vi "Navigation_Main_derping_stuff_up april 14_2.vi"() -> ()   [LabVIEW 2015]
uses:
  <vilib>/myRIO/Instrument Drivers/Onboard IO/PWM/typedefs/PWM Reference.ctl
  <vilib>/myRIO/Common/Instrument Driver Framework/Utilities/typedefs/myRIO Generic Hardware Reference.ctl
  <vilib>/myRIO/Common/Instrument Driver Framework/Utilities/typedefs/Hardware Version Enum.ctl
  <vilib>/myRIO/Common/Instrument Driver Framework/Utilities/typedefs/myRIO v1.0 Reference.ctl
  <vilib>/myRIO/Common/Instrument Driver Framework/Utilities/typedefs/Generic FPGA Reference.ctl
  <vilib>/myRIO/Common/Instrument Driver Framework/myRIO v1.0/PWM/typedefs/PWM Channels Enum.ctl
  <vilib>/myRIO/Instrument Drivers/Onboard IO/PWM/typedefs/PWM Configuration.ctl
  <vilib>/userdefined/High Color/nirio_resource_hc.ctl
  <vilib>/myRIO/Common/Instrument Driver Framework/myRIO v1.0/PWM/vis/myRIO v1.1 Open PWM.vi
  <vilib>/myRIO/Common/Instrument Driver Framework/Utilities/vis/Validate Channels.vi
  <vilib>/myRIO/Common/Instrument Driver Framework/myRIO v1.0/PWM/vis/myRIO v1.0 Reserve PWM.vi
  <vilib>/myRIO/Common/Instrument Driver Framework/myRIO v1.0/PWM/vis/myRIO v1.0 Build MUX Configuration PWM.vi
  <vilib>/myRIO/Common/Instrument Driver Framework/myRIO v1.0/Resource Manager/vis/myRIO v1.0 Reserve Channel List.vi
  <vilib>/myRIO/Common/Instrument Driver Framework/myRIO v1.0/Resource Manager/vis/myRIO v1.0 Create Configuration List.vi
  <vilib>/myRIO/Common/Instrument Driver Framework/myRIO v1.0/Resource Manager/vis/myRIO v1.0 Reserve Channel.vi
  <vilib>/myRIO/Common/Instrument Driver Framework/myRIO v1.0/Resource Manager/vis/myRIO v1.0 Unreserve Channel.vi
  <vilib>/myRIO/Common/Instrument Driver Framework/myRIO v1.0/Resource Manager/vis/myRIO v1.0 Build Mutex Name.vi
  <vilib>/FPGAPlugInAG/myRIO-1900/niLvFpga_Open_myRIO-1900.vi
  <vilib>/rvi/interface/common/dynamic/niFpgaDynamicAddResources.vi
  <vilib>/myRIO/Common/Instrument Driver Framework/Utilities/vis/FPGA Ref Manager.vi
  <vilib>/Utility/error.llb/Error Cluster From Error Code.vi
  <vilib>/myRIO/Common/Instrument Driver Framework/Utilities/vis/Ref Counter.vi
  <vilib>/rvi/errors/niLvFpgaAdjustHostInterfaceError.vi
  <vilib>/Utility/VariantDataType/GetNumericInfo.vi
  <vilib>/myRIO/Common/Instrument Driver Framework/myRIO v1.0/myRIO v1.1 Open.vi
  <vilib>/myRIO/Common/Instrument Driver Framework/Utilities/vis/IO Manager.vi
  <vilib>/myRIO/Common/Instrument Driver Framework/Utilities/vis/Configuration Manager.vi
  <vilib>/myRIO/Common/Instrument Driver Framework/myRIO v1.0/Resource Manager/vis/myRIO v1.0 Configure IO.vi
  <vilib>/myRIO/Common/Instrument Driver Framework/myRIO v1.0/myRIO v1.0 Close.vi
  <vilib>/myRIO/Common/Instrument Driver Framework/myRIO v1.0/PWM/vis/myRIO v1.0 Write PWM.vi
  <vilib>/addons/control/pid/pid.llb/PID (DBL).vi
  <vilib>/rvi/interface/nirviOpenFPGA/nirviOpenFPGA.xnode
  Navi/E/FPGA Bitfiles/NavigationProjec_FPGATarget2_FPGAMainNavigati_PWPHW8gwDxI.lvbitx
  <vilib>/rvi/interface/nirviReadWriteControl/nirviReadWriteControl.xnode
  <vilib>/myRIO/Instrument Drivers/Onboard IO/PWM/vis/myRIO PWM Open.xnode
  <vilib>/myRIO/Instrument Drivers/Onboard IO/PWM/PWM.lvlib
  <vilib>/myRIO/Instrument Drivers/Utilities/Utilities.lvlib
  NiFpgaLv.dll
  <vilib>/rvi/interface/Simulation/niFpgaSimulationCallBeginRW.vi
  <vilib>/addons/control/pid/NI_PID_pid.lvlib
panel:
  out "stop switch":dbl=1.0
  out "distance to goal":dbl
  out "loc_y":dbl
  out "loc_x":dbl
  out "loc_theta":dbl
  out "start y":dbl
  out "start angle":dbl=1.0
  out "start x":dbl=1.0
  in  "set start position":bool=TRUE
  out "goal reached":bool=TRUE
  out "x/y":dbl
  out "scale":dbl=1.0
  in  "x goal":dbl=10.0
  in  "L Desired Input Velocity (ft/s) 4":dbl(knob) scale=-4.0..4.0
  in  "R Min Linear Velocity (ft/s)  2":dbl=-2.0 format="%#_13g"
  in  "L Min Linear Velocity (ft/s) 9":dbl=-2.0 format="%#_13g"
  in  "R Max Linear Velocity (ft/s) 5":dbl=2.0 format="%#_13g"
  in  "L Max Linear Velocity (ft/s) 5":dbl=2.0 format="%#_13g"
  in  "R Desired Input Velocity (ft/s) 5":dbl(knob) scale=-4.0..4.0
  out "left":dbl
  out "right":dbl
  out "left wheels actual pwm":dbl
  in  "stop 3":bool
  out "left pwm":dbl(graph)
  out "dt out (s) 3":dbl format="%.3f"
  in  "output range 3":cluster{"output high":dbl, "output low":dbl}={"output high"=0.13333, "output low"=-0.13333} {"output low" format="%.6f"; "output high" format="%.5f"}
  in  "PID gains 3":T1={"proportional gain (Kc)"=0.002, "integral time (Ti, min)"=7e-07, "derivative time (Td, min)"=0.0} {"derivative time (Td, min)" format="%.8f"; "integral time (Ti, min)" format="%.8f"; "proportional gain (Kc)" format="%.8f"}
  out "desired pwm 2":dbl
  out "feedback 2":dbl
  out ".not. x? 3":bool
  out "Elapsed Time (s) 2":dbl caption="Elapsed Time (s)"
  out "x traveled 2":dbl
  out "y traveled 2":dbl
  out "avg 124":dbl
  out "avg 457":dbl
  out "psi dot 2":dbl
  out "distance traveled 2":dbl
  out "y dot 2":dbl
  out "x dot 2":dbl
  out "x position 2":dbl
  out "y position 2":dbl
  out "reset x y 2":dbl
  out "Tick Count(mSec) 2":u32 caption="Tick Count(mSec)"
  in  "start y 2":dbl=3.0
  in  "start x 2":dbl=1.0
  out "right wheels actual pwm":dbl
  in  "stop 2":bool
  out "right pwm":dbl(graph)
  out "dt out (s) 2":dbl format="%.3f"
  in  "output range 2":cluster{"output high":dbl, "output low":dbl}={"output high"=0.13333, "output low"=-0.13333} {"output low" format="%.6f"; "output high" format="%.5f"}
  in  "PID gains 2":T1={"proportional gain (Kc)"=0.002, "integral time (Ti, min)"=7e-07, "derivative time (Td, min)"=0.0} {"derivative time (Td, min)" format="%.8f"; "integral time (Ti, min)" format="%.8f"; "proportional gain (Kc)" format="%.8f"}
  out "desired pwm":dbl
  out "feedback":dbl
  out ".not. x? 2":bool
  out "Elapsed Time (s)":dbl
  out "LF Rot Velocity (rot/s)":dbl
  out "LM Rot Velocity (rot/s)":dbl
  out "LR Rot Velocity (rot/s)":dbl
  out "RR Rot Velocity (rot/s)":dbl
  out "RM Linear Velocity (rot/s)":dbl
  out "RF Linear Velocity (rot/s)":dbl
  in  "Encoder Reset":bool
  out "SYS.SELECTA":u8 format="%08b"
  out "ENC.B_c.CNTR":i32
  out "ENC.B_b.CNTR":i32
  out "ENC.B_a.CNTR":i32
  out "ENC.A_c.CNTR":i32
  out "ENC.A_b.CNTR":i32
  out "ENC.A_a.CNTR":i32
  in  "R Min Linear Velocity (ft/s)":dbl=-2.0 format="%#_13g"
  in  "R Max Linear Velocity (ft/s)":dbl=2.0 format="%#_13g"
  in  "L Min Linear Velocity (ft/s)":dbl=-2.0 format="%#_13g"
  in  "L Max Linear Velocity (ft/s)":dbl=2.0 format="%#_13g"
  out "Current Rot Velocity (rot/s)":T2(graph)
  # "Motor Control Parameters"
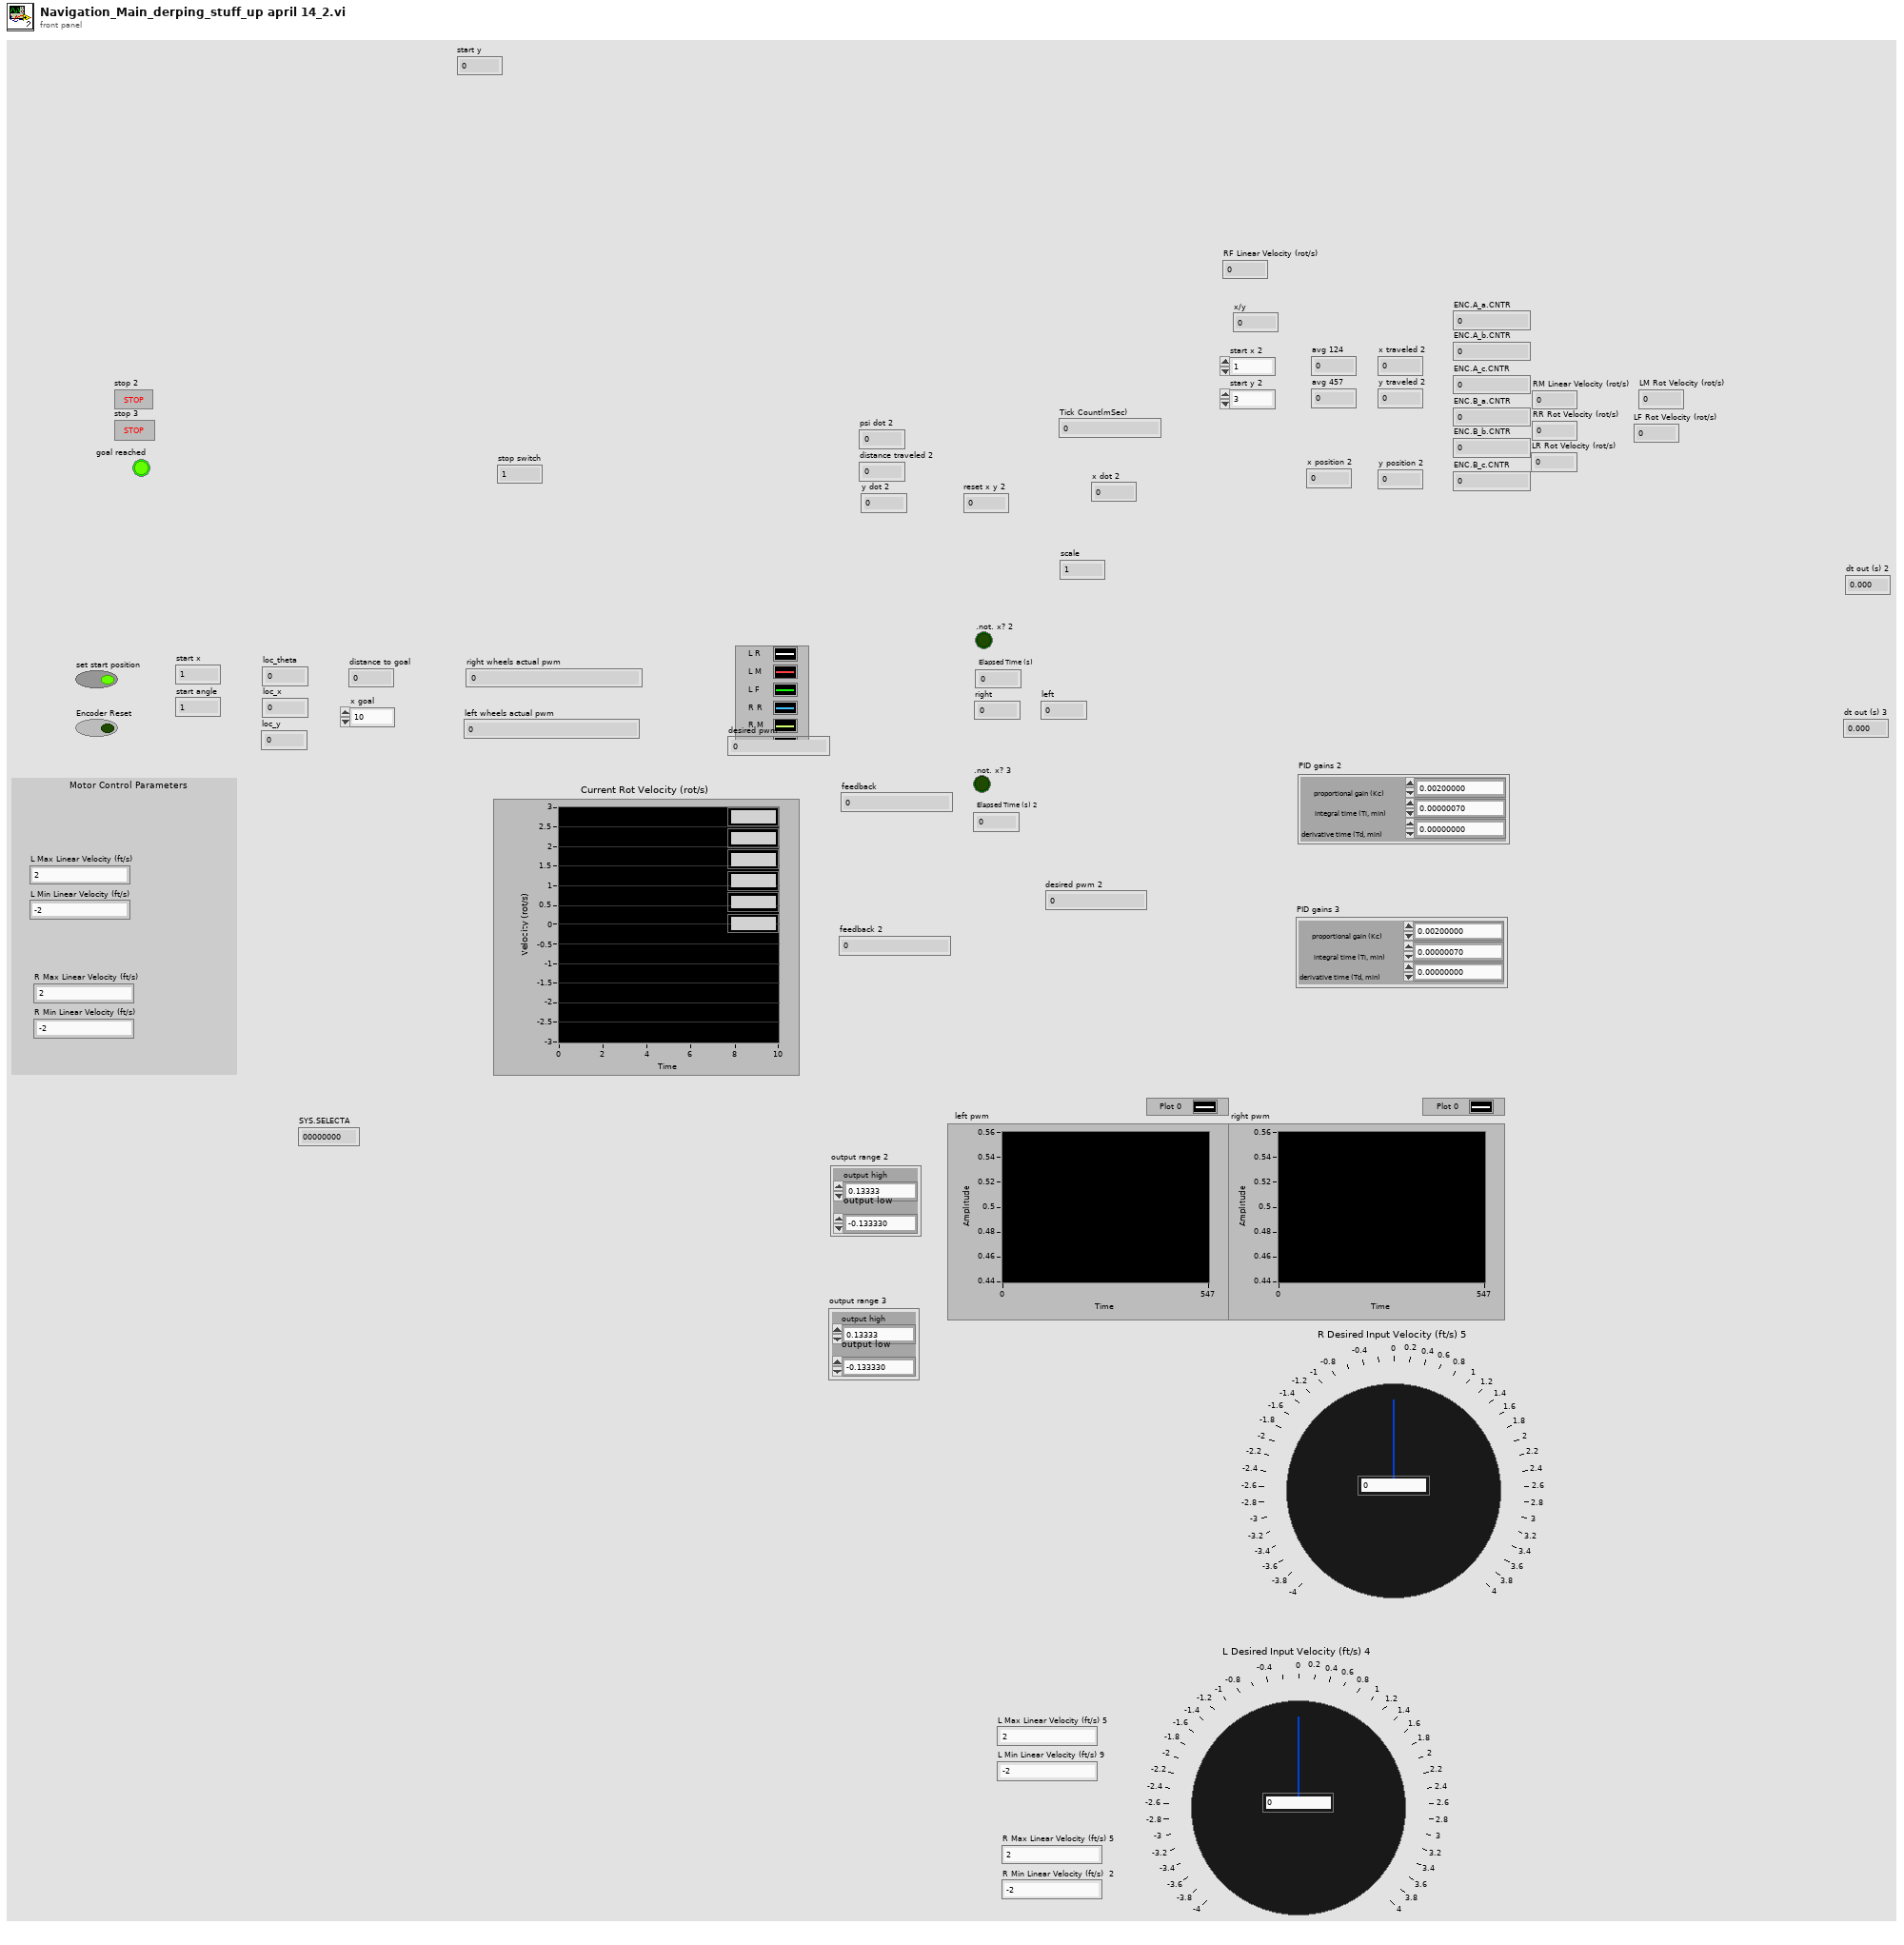
[diagram p1: front panel]
types:
  T1 = cluster{"proportional gain (Kc)":dbl, "integral time (Ti, min)":dbl, "derivative time (Td, min)":dbl}
  T2 = cluster{"Rotational Velocity (RPS)":dbl, "Rotational Velocity (RPS)":dbl, "Rotational Velocity (RPS)":dbl, "Rotational Velocity (RPS)":dbl, "Rotational Velocity (RPS)":dbl, "Rotational Velocity (RPS)":dbl}
  T3 = typedef "nirio_resource_hc.ctl" = tag
  T4 = typedef "Hardware Version Enum.ctl" = enum16{"Unknown", "myRIO-1900", "myRIO-1950", "roboRIO"}
  T5 = typedef "PWM.lvlib/PWM Reference.ctl" = cluster{"myRIO Reference":T6, "PWM Channels Enum":T9, "PWM Configuration":T10}
  T6 = typedef "myRIO Generic Hardware Reference.ctl" = cluster{"myRIO Model":T4, "myRIO Hardware Reference":T7}
  T7 = typedef "myRIO v1.0 Reference.ctl" = cluster{"Generic FPGA Reference":T8, "Allow multiple opens":bool}
  T8 = typedef "Generic FPGA Reference.ctl" = refnum<k20>
  T9 = typedef "PWM Channels Enum.ctl" = enum16{"Not Connected", "C/PWM0", "C/PWM1", "A/PWM0", "A/PWM1", "A/PWM2", "B/PWM0", "B/PWM1", "B/PWM2", "PWM/PWM0", "PWM/PWM1", "PWM/PWM2", "PWM/PWM3", "PWM/PWM4", "PWM/PWM5", "PWM/PWM6", "PWM/PWM7", "PWM/PWM8", "PWM/PWM9"}
  T10 = typedef "PWM.lvlib/PWM Configuration.ctl" = cluster{"Frequency":dbl, "Duty Cycle":dbl}
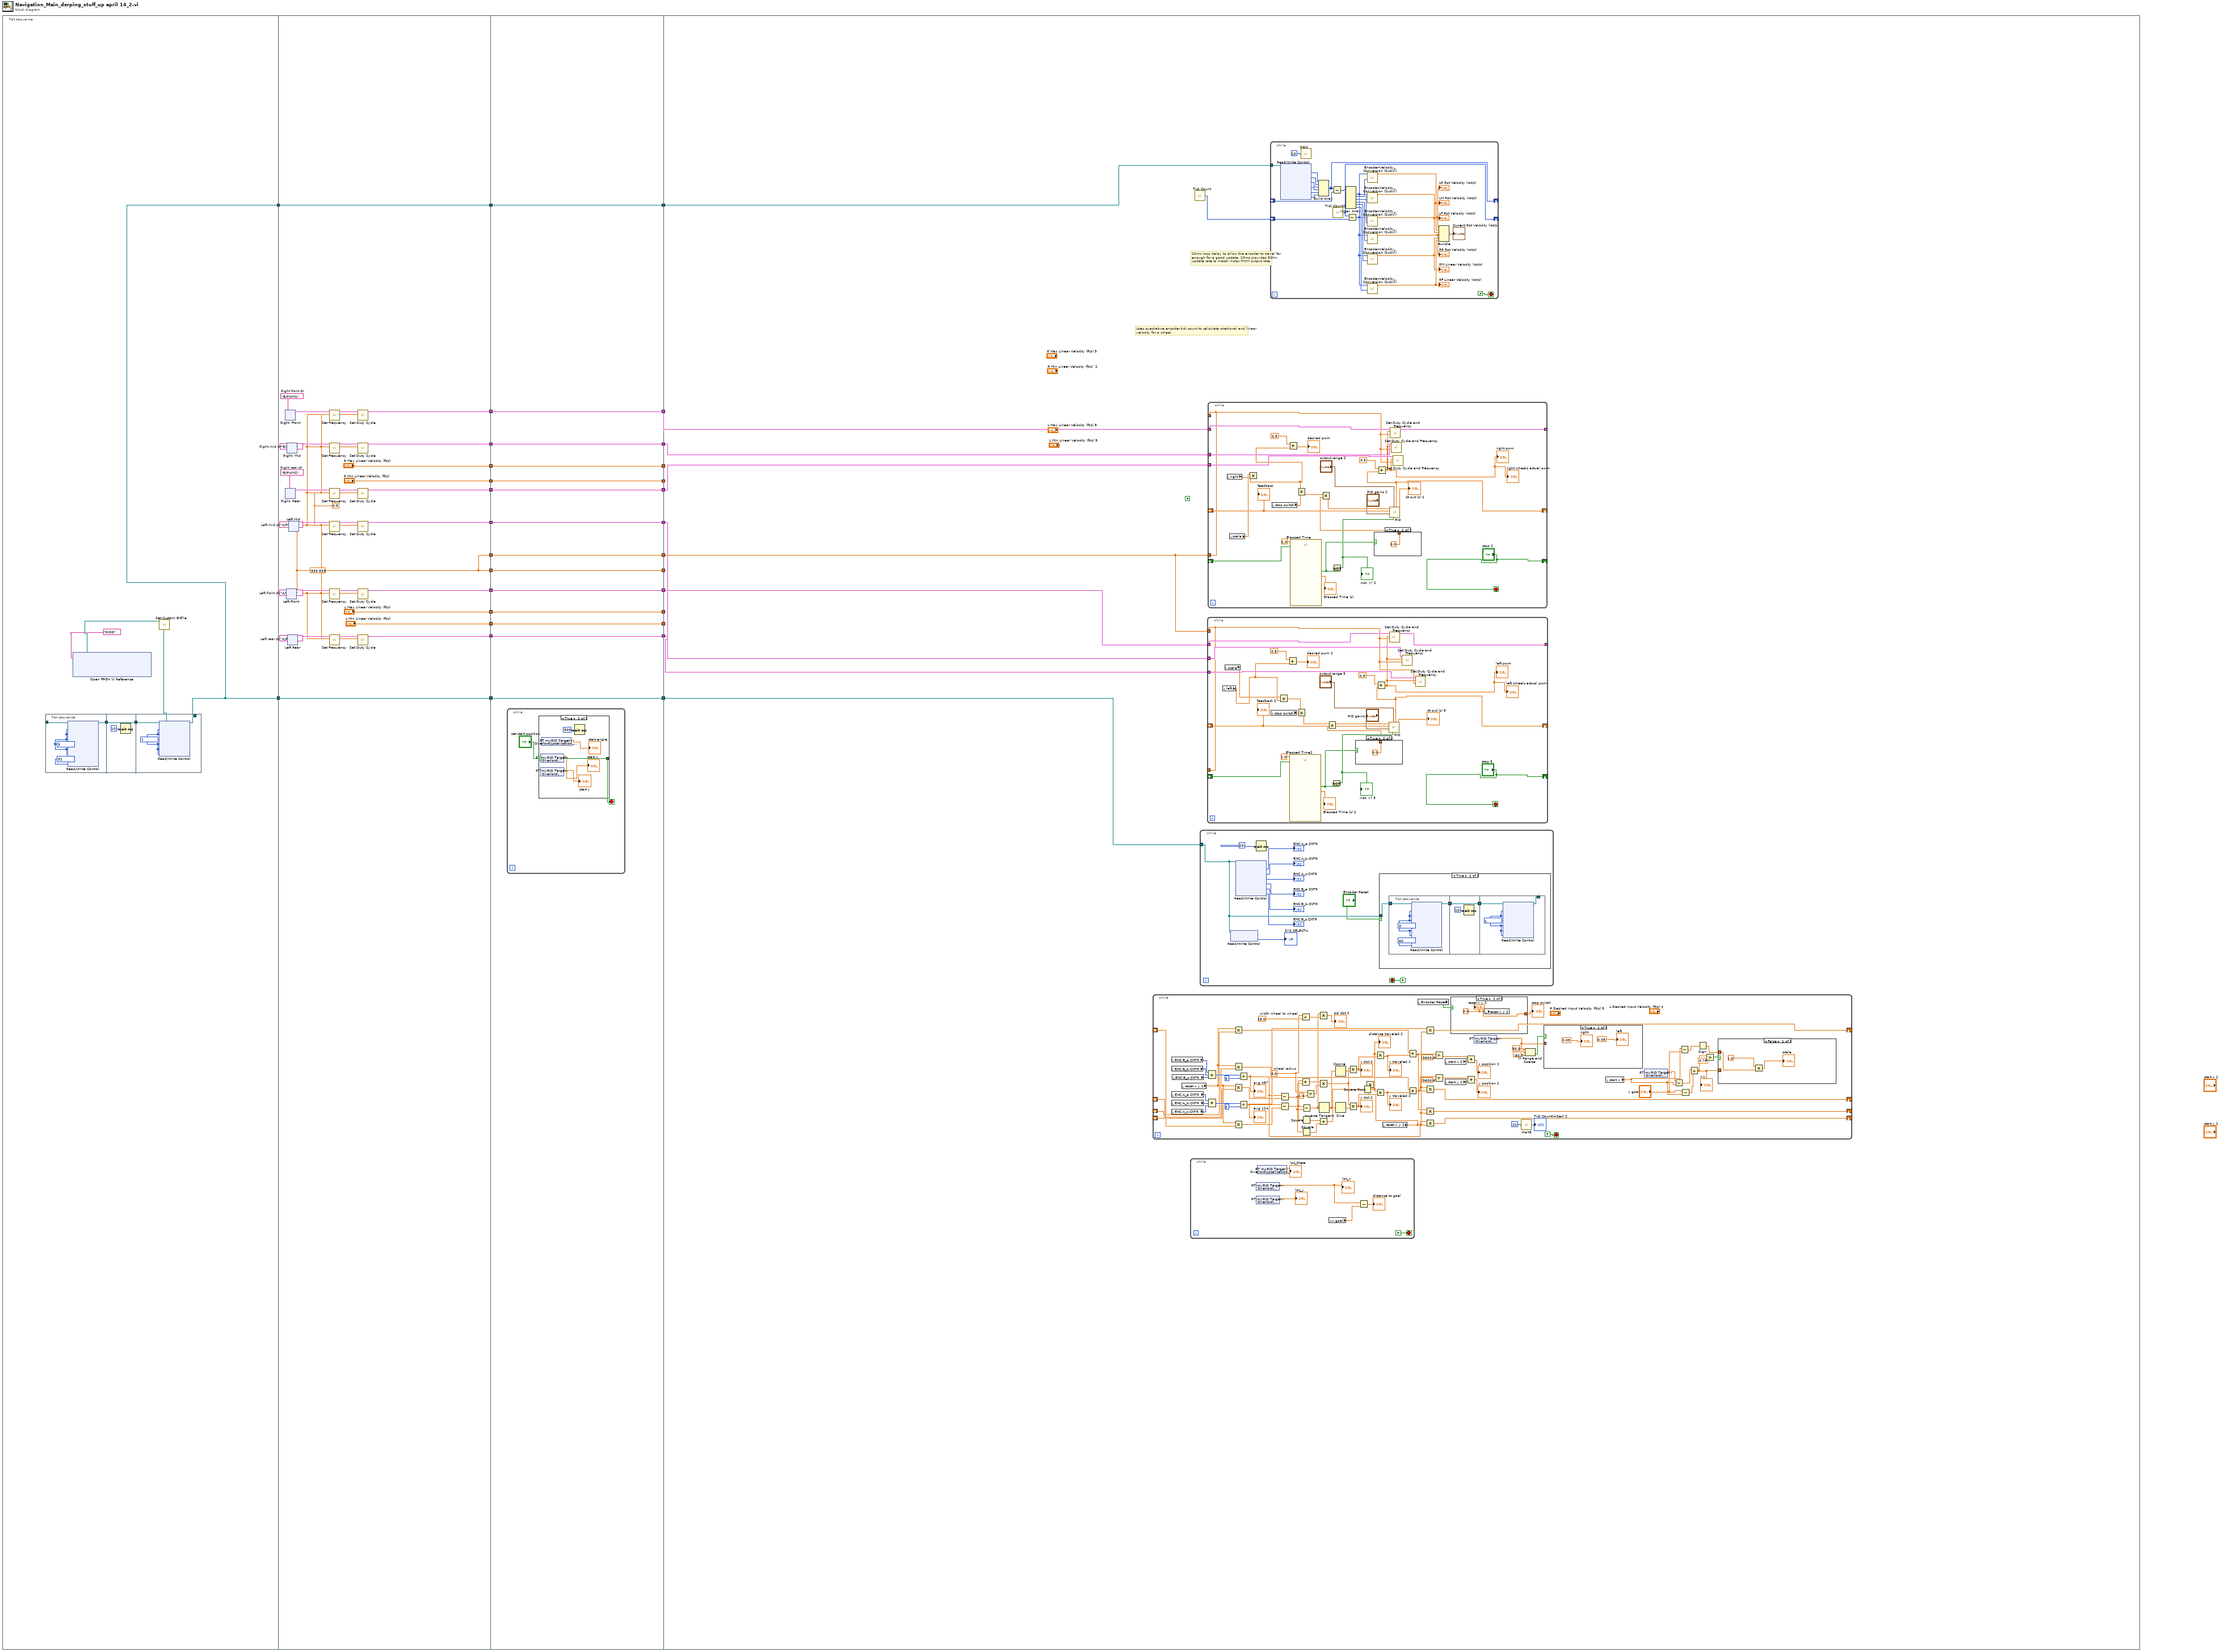
[diagram p0: block diagram]
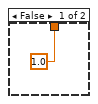
[diagram p3: hidden frame]
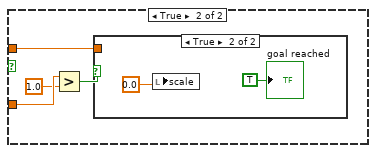
[diagram p4: hidden frame]
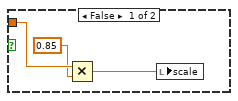
[diagram p5: hidden frame]
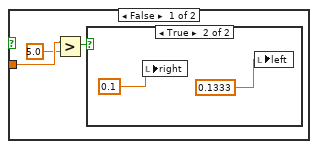
[diagram p6: hidden frame]
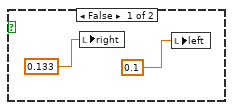
[diagram p7: hidden frame]
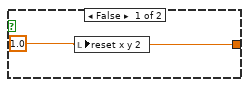
[diagram p8: hidden frame]
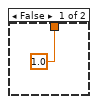
[diagram p9: hidden frame]
diagram:
  n1 = flat-sequence {
    tunnel: [w33] -> w30
    tunnel: [w33] -> w29
    tunnel: [w46] -> w28
    tunnel: [w61] -> w26
    tunnel: [w57] -> w24
    tunnel: [w56] -> w22
    tunnel: [w55] -> w20
    tunnel: [w54] -> w18
    tunnel: [w53] -> w16
    tunnel: ["L Max Linear Velocity (ft/s)"] -> w14
    tunnel: ["L Min Linear Velocity (ft/s)"] -> w12
    tunnel: ["R Max Linear Velocity (ft/s)"] -> w10
    tunnel: ["R Min Linear Velocity (ft/s)"] -> w8
    tunnel: [w48] -> w6
    tunnel: w30 -> [w47]
    tunnel: [w47] -> w4
    tunnel: w29 -> [w48]
    tunnel: [w46] -> w2
    tunnel: w28 -> [w187]
    tunnel: [w187] -> w27
    tunnel: w26 -> [w186]
    tunnel: [w186] -> w25
    tunnel: w24 -> [w185]
    tunnel: [w185] -> w23
    tunnel: w22 -> [w184]
    tunnel: [w184] -> w21
    tunnel: w20 -> [w183]
    tunnel: [w183] -> w19
    tunnel: w18 -> [w182]
    tunnel: [w182] -> w17
    tunnel: w16 -> [w181]
    tunnel: [w181] -> w15
    tunnel: w14 -> [w180]
    tunnel: [w180] -> w13
    tunnel: w12 -> [w179]
    tunnel: [w179] -> w11
    tunnel: w10 -> [w178]
    tunnel: [w178] -> w9
    tunnel: w8 -> [w177]
    tunnel: [w177] -> w7
    tunnel: w6 -> [w176]
    tunnel: [w176] -> w5
    tunnel: w4 -> [w175]
    tunnel: [w175] -> w3
    tunnel: w2 -> [w174]
    tunnel: [w174] -> w1
    tunnel: w27 -> [_]
    tunnel: w25 -> [w195]
    tunnel: w23 -> [w201]
    tunnel: w21 -> [w198]
    tunnel: w19 -> [w197]
    tunnel: w17 -> [w196]
    tunnel: w15 -> [w200]
    tunnel: w13 -> [_]
    tunnel: w11 -> [_]
    tunnel: w9 -> [_]
    tunnel: w7 -> [_]
    tunnel: w5 -> [w203]
    tunnel: w3 -> [w202]
    tunnel: w1 -> [w199]
    frame #0 {
      n2 = flat-sequence {
        tunnel: w34 -> [w39]
        tunnel: [w37] -> w36
        tunnel: w36 -> [w41]
        tunnel: [w41] -> w35
        tunnel: w35 -> [w44]
        tunnel: [w43] -> w33
        frame #0 {
          w38 = u8 32 ("SYS.SELECTA")
          w40 = u8 3 ("ENC.B_c.CNFG")
          n3 = xnode "Read/Write Control"("FPGA VI Reference In"=w39, "ENC.A_a.CNFG"=w40, "ENC.A_b.CNFG"=w40, "ENC.A_c.CNFG"=w40, "ENC.B_a.CNFG"=w40, "ENC.B_b.CNFG"=w40, "ENC.B_c.CNFG"=w40, "SYS.SELECTA"=w38, "SYS.SELECTB"=w38) -> ("FPGA VI Reference Out"=w37:refnum<k20>)  [unwired: 1 in, 1 out]
        }
        frame #1 {
          n4 = Wait (ms)(milliseconds to wait=u32 10) -> ()  [unwired: 1 out]
        }
        frame #2 {
          w45 = u8 1 ("ENC.B_c.CNFG")
          n5 = xnode "Read/Write Control"("FPGA VI Reference In"=w44, "ENC.A_a.CNFG"=w45, "ENC.A_b.CNFG"=w45, "ENC.A_c.CNFG"=w45, "ENC.B_a.CNFG"=w45, "ENC.B_b.CNFG"=w45, "ENC.B_c.CNFG"=w45) -> ("FPGA VI Reference Out"=w43:refnum<k20>)  [unwired: 1 in, 1 out]
        }
      }
      n6 = xnode "Open FPGA VI Reference"("resource name"=tag "RIO0") -> ("FPGA VI Reference Out"=w32:refnum<k20>)  [unwired: 1 in, 1 out]
      n7 = call <vilib>:"Set Custom Bitfile.vi"("Custom FPGA Reference In"=w32) -> ("Custom FPGA Reference Out"=w34:refnum<k20>)  [unwired: 9 in, 1 out]
    }
    frame #1 {
      w58 = 0.5 ("Duty Cycle")
      w46 = 333.333 ("Frequency [Hz]")
      w72 = tag "B/PWM2"  # Right rear ch
      w73 = tag "B/PWM0"  # Right mid ch
      w74 = tag "B/PWM1"  # Right front ch
      w75 = tag "A/PWM2"  # Left rear ch
      w76 = tag "A/PWM1"  # Left mid ch
      w77 = tag "A/PWM0"  # Left front ch
      n8 = xnode "Right  Front"("Channel Name"=w74) -> ("PWM Ref Out"=w68:T5)  [unwired: 2 in, 1 out]
      n9 = xnode "Right  Rear"("Channel Name"=w72) -> ("PWM Ref Out"=w66:T5)  [unwired: 2 in, 1 out]
      n10 = xnode "Left Front"("Channel Name"=w77) -> ("PWM Ref Out"=w71:T5)  [unwired: 2 in, 1 out]
      n11 = xnode "Right  Mid"("Channel Name"=w73) -> ("PWM Ref Out"=w67:T5)  [unwired: 2 in, 1 out]
      n12 = xnode "Left Rear"("Channel Name"=w75) -> ("PWM Ref Out"=w69:T5)  [unwired: 2 in, 1 out]
      n13 = xnode "Left Mid"("Channel Name"=w76) -> ("PWM Ref Out"=w70:T5)  [unwired: 2 in, 1 out]
      n14 = call <vilib>:"Set Frequency.vi"("Frequency [Hz]"=w46, "PWM Ref In"=w68) -> ("PWM Ref Out"=w62:T5)  [unwired: 7 in, 1 out]
      n15 = call <vilib>:"Set Frequency.vi"("Frequency [Hz]"=w46, "PWM Ref In"=w67) -> ("PWM Ref Out"=w63:T5)  [unwired: 7 in, 1 out]
      n16 = call <vilib>:"Set Frequency.vi"("Frequency [Hz]"=w46, "PWM Ref In"=w66) -> ("PWM Ref Out"=w64:T5)  [unwired: 7 in, 1 out]
      n17 = call <vilib>:"Set Frequency.vi"("Frequency [Hz]"=w46, "PWM Ref In"=w70) -> ("PWM Ref Out"=w59:T5)  [unwired: 7 in, 1 out]
      n18 = call <vilib>:"Set Frequency.vi"("Frequency [Hz]"=w46, "PWM Ref In"=w71) -> ("PWM Ref Out"=w65:T5)  [unwired: 7 in, 1 out]
      n19 = call <vilib>:"Set Frequency.vi"("Frequency [Hz]"=w46, "PWM Ref In"=w69) -> ("PWM Ref Out"=w60:T5)  [unwired: 7 in, 1 out]
      n20 = call <vilib>:"Set Duty Cycle.vi"("Duty Cycle"=w58, "PWM Ref In"=w62) -> ("PWM Ref Out"=w57:T5)  [unwired: 7 in, 1 out]
      n21 = call <vilib>:"Set Duty Cycle.vi"("Duty Cycle"=w58, "PWM Ref In"=w63) -> ("PWM Ref Out"=w56:T5)  [unwired: 7 in, 1 out]
      n22 = call <vilib>:"Set Duty Cycle.vi"("Duty Cycle"=w58, "PWM Ref In"=w64) -> ("PWM Ref Out"=w55:T5)  [unwired: 7 in, 1 out]
      n23 = call <vilib>:"Set Duty Cycle.vi"("Duty Cycle"=w58, "PWM Ref In"=w59) -> ("PWM Ref Out"=w54:T5)  [unwired: 7 in, 1 out]
      n24 = call <vilib>:"Set Duty Cycle.vi"("Duty Cycle"=w58, "PWM Ref In"=w65) -> ("PWM Ref Out"=w53:T5)  [unwired: 7 in, 1 out]
      n25 = call <vilib>:"Set Duty Cycle.vi"("Duty Cycle"=w58, "PWM Ref In"=w60) -> ("PWM Ref Out"=w61:T5)  [unwired: 7 in, 1 out]
    }
    frame #2 {
      n26 = while {
        stop <- w188 stop-if-true
        n27 = case shown="True" "set start position" {
          selector: "set start position" -> [_ w194]
          tunnel: [_ w194] -> w188
          frame False {
          }
          frame True {
            n28 = shared-variable "RT myRIO Target - Overlord\\Localization_Variables_r0.lvlib\\loc_x"() -> (→"start x":dbl)  [unwired: 1 in, 1 out]
            n29 = shared-variable "RT myRIO Target - Overlord\\Localization_Variables_r0.lvlib\\loc_y"() -> (→"start y":dbl)  [unwired: 1 in, 1 out]
            n30 = shared-variable "RT myRIO Target - Overlord\\Localization_Variables_r0.lvlib\\loc_theta"() -> (→"start angle":dbl)  [unwired: 1 in, 1 out]
            n31 = Wait (ms)(milliseconds to wait=u32 500) -> ()  [unwired: 1 out]
          }
        }
      }
    }
    frame #3 {
      (unwired) FALSE
      # "Uses quadrature encoder tick count to calculate rotational and linear velocity for a wheel."
      # "20ms loop delay to allow the encoder to travel far enough for a good update. 20ms provides 50Hz update rate to match motor PWM output rate."
      n32 = while {
        shift-right: [w266] -> _
        shift-left: _ -> [w304]
        shift-right: [w263] -> _
        shift-left: _ -> [w303]
        shift-right: [w265] -> _
        shift-left: _ -> [w278]
        shift-right: [w264] -> _
        shift-left: _ -> [w277]
        stop <- FALSE stop-if-true
        w299 = 28.0  # width wheel to wheel
        w300 = 4.0  # wheel radius
        n33 = local read "ENC.B_a.CNTR"() -> (w309:i32)
        n34 = local read "ENC.B_b.CNTR"() -> (w308:i32)
        n35 = local read "ENC.A_a.CNTR"() -> (w312:i32)
        n36 = local read "ENC.A_b.CNTR"() -> (w311:i32)
        n37 = local read "ENC.A_c.CNTR"() -> (w310:i32)
        n38 = local read "ENC.B_c.CNTR"() -> (w307:i32)
        n39 = local read "reset x y 2"() -> (w262:dbl)
        n40 = Compound Arithmetic op=ADD(w309, w308, w307) -> (w315:i32)
        n41 = Compound Arithmetic op=ADD(w312, w311, w310) -> (w316:i32)
        n42 = Multiply(x=w262, y=w277) -> (x*y=w268:dbl)
        n43 = Multiply(x=w262, y=w278) -> (x*y=w269:dbl)
        n44 = Multiply(x=w262, y=w303) -> (x*y=w267:dbl)
        n45 = Multiply(x=w262, y=w304) -> (x*y=w270:dbl)
        n46 = Divide(x=w315, y=3) -> (x/y=w302:dbl)
        "avg 457" <- w302
        n47 = Divide(x=w316, y=3) -> (x/y=w305:dbl)
        "avg 124" <- w305
        n48 = Subtract(x=w302, y=w267) -> (x-y=w292:dbl)
        n49 = Subtract(x=w305, y=w270) -> (x-y=w293:dbl)
        n50 = Divide(x=w300, y=w299) -> (x/y=w295:dbl)
        n51 = Add(x=w293, y=w292) -> (x+y=w297:dbl)
        n52 = Square(x=w293) -> (x^2=w290:dbl)
        n53 = Square(x=w292) -> (x^2=w291:dbl)
        n54 = Subtract(x=w293, y=w292) -> (x-y=w296:dbl)
        n55 = Divide(x=w300, y=2.0) -> (x/y=w298:dbl)
        n56 = Multiply(x=w296, y=w295) -> (x*y=→"psi dot 2":dbl)
        n57 = Multiply(x=w297, y=w298) -> (x*y=w286:dbl)
        n58 = Add(x=w290, y=w291) -> (x+y=w289:dbl)
        n59 = Inverse Tangent(1:w296) -> (0:w294:dbl)
        n60 = Cosine(x=w294) -> (cos(x)=w287:dbl)
        n61 = Sine(x=w294) -> (sin(x)=w288:dbl)
        n62 = Multiply(x=w286, y=w287) -> (x*y=w284:dbl)
        "x dot 2" <- w284
        n63 = Multiply(x=w286, y=w288) -> (x*y=w285:dbl)
        "y dot 2" <- w285
        n64 = Square Root(x=w289) -> (sqrt(x)=w283:dbl)
        n65 = local read "reset x y 2"() -> (w260:dbl)
        n66 = Multiply(x=w283, y=w260) -> (x*y=w261:dbl)
        "distance traveled 2" <- w261
        n67 = Multiply(x=w261, y=w284) -> (x*y=w282:dbl)
        "x traveled 2" <- w282
        n68 = Multiply(x=w261, y=w285) -> (x*y=w281:dbl)
        "y traveled 2" <- w281
        n69 = Add(x=w268, y=w282) -> (x+y=w280:dbl)
        n70 = Add(x=w269, y=w281) -> (x+y=w272:dbl)
        n71 = local read "Encoder Reset"() -> (w259:bool)
        n72 = Multiply(x=w305, y=w260) -> (x*y=w266:dbl)
        n73 = Multiply(x=w260, y=w272) -> (x*y=w265:dbl)
        n74 = Multiply(x=w280, y=w260) -> (x*y=w264:dbl)
        n75 = Multiply(x=w302, y=w260) -> (x*y=w263:dbl)
        n76 = Divide(x=w280, y=9600.0) -> (x/y=w275:dbl)
        n77 = Divide(x=w272, y=9600.0) -> (x/y=w276:dbl)
        n78 = local read "start x 2"() -> (w273:dbl)
        n79 = local read "start y 2"() -> (w274:dbl)
        n80 = case shown="True" w259 {
          tunnel: [w339 w340] -> w240
          frame False {
            w339 = 1.0
            n81 = local write "reset x y 2"(w339) -> ()
          }
          frame True {
            w340 = 0.0
            n82 = local write "reset x y 2"(w340) -> ()
            "reset x y 2" <- w340
          }
        }
        "stop switch" <- w240
        n83 = Add(x=w275, y=w273) -> (x+y=→"x position 2":dbl)
        n84 = Add(x=w276, y=w274) -> (x+y=→"y position 2":dbl)
        n85 = shared-variable "RT myRIO Target - Overlord\\Localization_Variables_r0.lvlib\\loc_x"() -> (w242:dbl)  [unwired: 1 in, 1 out]
        n86 = call "Wait3"("Count(mSec)"=u32 20) -> ("Tick Count(mSec)"=→"Tick Count(mSec) 2":u32)
        n87 = In Range and Coerce(upper limit=50.0, x=w242, lower limit=-50.0) -> (In Range?=w253:bool)  [unwired: 1 out]
        n88 = case shown="True" w253 {
          tunnel: w242 -> [w332 _]
          frame False {
            n89 = Greater?(x=w332, y=5.0) -> (0:w330:bool)
            n90 = case shown="True" w330 {
              frame False {
                n91 = local write "right"(0.133) -> ()
                n92 = local write "left"(0.1) -> ()
              }
              frame True {
                n93 = local write "right"(0.1) -> ()
                n94 = local write "left"(0.1333) -> ()
              }
            }
          }
          frame True {
            "right" <- 0.05
            "left" <- 0.05
          }
        }
        n95 = local read "start x"() -> (w244:dbl)
        n96 = shared-variable "RT myRIO Target - Overlord\\Localization_Variables_r0.lvlib\\loc_x"() -> (w241:dbl)  [unwired: 1 in, 1 out]
        n97 = Subtract(x=w241, y=w244) -> (x-y=w249:dbl)
        n98 = Subtract(x=w244, y="x goal") -> (x-y=w246:dbl)
        n99 = Subtract(x="x goal", y=w244) -> (x-y=w248:dbl)
        n100 = Divide(x=w249, y=w248) -> (x/y=w250:dbl)
        "x/y" <- w250
        n101 = Sign(1:w246) -> (0:w245:dbl)
        n102 = Greater?(x=w250, y=0.75) -> (0:w251:bool)
        n103 = case shown="False" w251 {
          tunnel: w250 -> [_ w324]
          tunnel: w245 -> [w319 w321]
          frame False {
            n104 = Multiply(x=1.0, y=w319) -> (x*y=→"scale":dbl)
          }
          frame True {
            n105 = Greater?(x=w324, y=1.0) -> (0:w322:bool)
            n106 = case shown="True" w322 {
              tunnel: w321 -> [w327 _]
              frame False {
                n107 = Multiply(x=w327, y=0.85) -> (x*y=w325:dbl)
                n108 = local write "scale"(w325) -> ()
              }
              frame True {
                n109 = local write "scale"(0.0) -> ()
                "goal reached" <- TRUE
              }
            }
          }
        }
      }
      n110 = while {
        stop <- FALSE stop-if-true
        n111 = shared-variable "RT myRIO Target - Overlord\\Localization_Variables_r0.lvlib\\loc_x"() -> (w208:dbl)  [unwired: 1 in, 1 out]
        "loc_x" <- w208
        n112 = shared-variable "RT myRIO Target - Overlord\\Localization_Variables_r0.lvlib\\loc_y"() -> (→"loc_y":dbl)  [unwired: 1 in, 1 out]
        n113 = shared-variable "RT myRIO Target - Overlord\\Localization_Variables_r0.lvlib\\loc_theta"() -> (→"loc_theta":dbl)  [unwired: 1 in, 1 out]
        n114 = local read "x goal"() -> (w207:dbl)
        n115 = Subtract(x=w208, y=w207) -> (x-y=→"distance to goal":dbl)
      }
      n116 = call "Tick Count"() -> ("Tick Count(uSec)"=w204:u32)
      n117 = while {
        tunnel: w203 -> [w370]
        stop <- FALSE stop-if-true
        n118 = xnode "Read/Write Control"("FPGA VI Reference In"=w370) -> ("SYS.SELECTA"=→"SYS.SELECTA":u8)  [unwired: 1 in, 2 out]
        n119 = xnode "Read/Write Control"("FPGA VI Reference In"=w370) -> ("ENC.A_a.CNTR"=→"ENC.A_a.CNTR":u32, "ENC.A_b.CNTR"=→"ENC.A_b.CNTR":u32, "ENC.A_c.CNTR"=→"ENC.A_c.CNTR":u32, "ENC.B_a.CNTR"=→"ENC.B_a.CNTR":u32, "ENC.B_b.CNTR"=→"ENC.B_b.CNTR":u32, "ENC.B_c.CNTR"=→"ENC.B_c.CNTR":u32)  [unwired: 1 in, 2 out]
        n120 = Wait (ms)(milliseconds to wait=u32 20) -> ()  [unwired: 1 out]
        n121 = case shown="True" "Encoder Reset" {
          tunnel: w370 -> [_ w381]
          frame False {
          }
          frame True {
            n122 = flat-sequence {
              tunnel: w381 -> [w386]
              tunnel: [w384] -> w383
              tunnel: w383 -> [w388]
              tunnel: [w388] -> w382
              tunnel: w382 -> [w391]
              tunnel: [w390] -> _
              frame #0 {
                w385 = u8 60 ("SYS.SELECTA")
                w387 = u8 3 ("ENC.B_c.CNFG")
                n123 = xnode "Read/Write Control"("FPGA VI Reference In"=w386, "ENC.A_a.CNFG"=w387, "ENC.A_b.CNFG"=w387, "ENC.A_c.CNFG"=w387, "ENC.B_a.CNFG"=w387, "ENC.B_b.CNFG"=w387, "ENC.B_c.CNFG"=w387, "SYS.SELECTA"=w385, "SYS.SELECTB"=w385) -> ("FPGA VI Reference Out"=w384:refnum<k20>)  [unwired: 1 in, 1 out]
              }
              frame #1 {
                n124 = Wait (ms)(milliseconds to wait=u32 10) -> ()  [unwired: 1 out]
              }
              frame #2 {
                w392 = u8 1 ("ENC.B_c.CNFG")
                n125 = xnode "Read/Write Control"("FPGA VI Reference In"=w391, "ENC.A_a.CNFG"=w392, "ENC.A_b.CNFG"=w392, "ENC.A_c.CNFG"=w392, "ENC.B_a.CNFG"=w392, "ENC.B_b.CNFG"=w392, "ENC.B_c.CNFG"=w392) -> ("FPGA VI Reference Out"=w390:refnum<k20>)  [unwired: 1 in, 1 out]
              }
            }
          }
        }
      }
      n126 = while {
        tunnel: w200 -> [w236]
        tunnel: [w237] -> _
        tunnel: w199 -> [w220]
        shift-right: [w219] -> _
        shift-left: _ -> [w232]
        shift-right: ["stop 3"] -> _
        shift-left: _ -> [w228]
        tunnel: [w220] -> _
        tunnel: w196 -> [w223]
        tunnel: w195 -> [w222]
        stop <- "stop 3" stop-if-true
        n127 = local read "left"() -> (w218:dbl)
        n128 = local read "scale"() -> (w224:dbl)
        n129 = local read "stop switch"() -> (w215:dbl)
        n130 = Multiply(x=w224, y=w218) -> (x*y=w217:dbl)
        n131 = Add(x=0.5, y=w218) -> (x+y=→"desired pwm 2":dbl)
        n132 = call "Elapsed Time2"("Time Target (s)"=2.0, "Reset"=w228) -> ("Elapsed Time (s)"=→"Elapsed Time (s) 2":dbl, "Time has Elapsed"=w213:bool)  [unwired: 10 in, 6 out]
        n133 = Multiply(x=w217, y=w215) -> (x*y=w216:dbl)
        n134 = Not(x=w213) -> (.not. x?=w230:bool)
        ".not. x? 3" <- w230
        n135 = case shown="True" w213 {
          tunnel: [1.0 0.0] -> w211
          frame False {
          }
          frame True {
          }
        }
        n136 = Multiply(x=w216, y=w211) -> (x*y=w212:dbl)
        n137 = call-poly <vilib>:"PID.vi"("reinitialize? (F)"=w230, "output range"="output range 3", "PID gains"="PID gains 3", "process variable"=w232, "setpoint"=w212) -> ("dt out (s)"=→"dt out (s) 3":dbl, "output"=w219:dbl)  [unwired: 5 in]
        n138 = Add(x=0.5, y=w219) -> (x+y=w221:dbl)
        "left wheels actual pwm" <- w221
        "left pwm" <- w221
        n139 = call <vilib>:"Set Duty Cycle and Frequency.vi"("Frequency [Hz]"=w220, "Duty Cycle"=w221, "PWM Ref In"=w236) -> ("PWM Ref Out"=w237:T5)  [unwired: 6 in, 1 out]
        n140 = call <vilib>:"Set Duty Cycle and Frequency.vi"("Frequency [Hz]"=w220, "Duty Cycle"=w221, "PWM Ref In"=w223) -> ()  [unwired: 6 in, 2 out]
        n141 = call <vilib>:"Set Duty Cycle and Frequency.vi"("Frequency [Hz]"=w220, "Duty Cycle"=w221, "PWM Ref In"=w222) -> ()  [unwired: 6 in, 2 out]
        "feedback 2" <- w232
      }
      n142 = while {
        tunnel: w201 -> [w366]
        tunnel: [w367] -> _
        tunnel: [w350] -> _
        shift-right: [w349] -> _
        shift-left: _ -> [w362]
        shift-right: ["stop 2"] -> _
        shift-left: _ -> [w358]
        tunnel: w199 -> [w350]
        tunnel: w198 -> [w353]
        tunnel: w197 -> [w352]
        stop <- "stop 2" stop-if-true
        n143 = local read "right"() -> (w348:dbl)
        n144 = local read "scale"() -> (w354:dbl)
        n145 = Multiply(x=w354, y=w348) -> (x*y=w347:dbl)
        n146 = local read "stop switch"() -> (w345:dbl)
        n147 = Add(x=0.5, y=w347) -> (x+y=→"desired pwm":dbl)
        n148 = call "Elapsed Time"("Time Target (s)"=2.0, "Reset"=w358) -> ("Elapsed Time (s)"=→"Elapsed Time (s)":dbl, "Time has Elapsed"=w343:bool)  [unwired: 10 in, 6 out]
        n149 = Multiply(x=w347, y=w345) -> (x*y=w346:dbl)
        n150 = Not(x=w343) -> (.not. x?=w360:bool)
        ".not. x? 2" <- w360
        n151 = case shown="True" w343 {
          tunnel: [1.0 0.0] -> w341
          frame False {
          }
          frame True {
          }
        }
        n152 = Multiply(x=w346, y=w341) -> (x*y=w342:dbl)
        n153 = call-poly <vilib>:"PID.vi"("reinitialize? (F)"=w360, "output range"="output range 2", "PID gains"="PID gains 2", "process variable"=w362, "setpoint"=w342) -> ("dt out (s)"=→"dt out (s) 2":dbl, "output"=w349:dbl)  [unwired: 5 in]
        n154 = Add(x=0.5, y=w349) -> (x+y=w351:dbl)
        "right wheels actual pwm" <- w351
        "right pwm" <- w351
        n155 = call <vilib>:"Set Duty Cycle and Frequency.vi"("Frequency [Hz]"=w350, "Duty Cycle"=w351, "PWM Ref In"=w366) -> ("PWM Ref Out"=w367:T5)  [unwired: 6 in, 1 out]
        n156 = call <vilib>:"Set Duty Cycle and Frequency.vi"("Frequency [Hz]"=w350, "Duty Cycle"=w351, "PWM Ref In"=w353) -> ()  [unwired: 6 in, 2 out]
        n157 = call <vilib>:"Set Duty Cycle and Frequency.vi"("Frequency [Hz]"=w350, "Duty Cycle"=w351, "PWM Ref In"=w352) -> ()  [unwired: 6 in, 2 out]
        "feedback" <- w362
      }
      n158 = while {
        shift-right: [w411] -> _
        shift-left: _ -> [w410]
        shift-right: [w408] -> _
        shift-left: w204 -> [w407]
        tunnel: w202 -> [w418]
        stop <- FALSE stop-if-true
        n159 = xnode "Read/Write Control"("FPGA VI Reference In"=w418) -> ("ENC.A_a.CNTR"=w417:u32, "ENC.A_b.CNTR"=w416:u32, "ENC.A_c.CNTR"=w415:u32, "ENC.B_a.CNTR"=w414:u32, "ENC.B_b.CNTR"=w413:u32, "ENC.B_c.CNTR"=w412:u32)  [unwired: 1 in, 2 out]
        n160 = call "Wait"("Count(mSec)"=u32 20) -> ()  [unwired: 1 out]
        n161 = Build Array(w417, w416, w415, w414, w413, w412) -> (w411:u32[])
        n162 = Subtract(x=w411, y=w410) -> (x-y=w409:u32[])
        n163 = call "Tick Count2"() -> ("Tick Count(uSec)"=w408:u32)
        n164 = Index Array(array=w409) -> (element #1=w406:u32, element #2=w405:u32, element #3=w404:u32, element #4=w403:u32, element #5=w402:u32, element #6=w401:u32)  [unwired: 6 in]
        n165 = Subtract(x=w408, y=w407) -> (x-y=w400:u32)
        n166 = call "Encoder-Velocity_Conversion (SubVI).vi"("delta  Encoder Count"=w405, "dt (uSec)"=w400) -> ("Rotational Velocity (RPS)"=w395:dbl)  [unwired: 7 in, 2 out]
        "LM Rot Velocity (rot/s)" <- w395
        n167 = call "Encoder-Velocity_Conversion (SubVI).vi"("delta  Encoder Count"=w404, "dt (uSec)"=w400) -> ("Rotational Velocity (RPS)"=w394:dbl)  [unwired: 7 in, 2 out]
        "LF Rot Velocity (rot/s)" <- w394
        n168 = call "Encoder-Velocity_Conversion (SubVI).vi"("delta  Encoder Count"=w406, "dt (uSec)"=w400) -> ("Rotational Velocity (RPS)"=w396:dbl)  [unwired: 7 in, 2 out]
        "LR Rot Velocity (rot/s)" <- w396
        n169 = call "Encoder-Velocity_Conversion (SubVI).vi"("delta  Encoder Count"=w403, "dt (uSec)"=w400) -> ("Rotational Velocity (RPS)"=w393:dbl)  [unwired: 7 in, 2 out]
        "RR Rot Velocity (rot/s)" <- w393
        n170 = call "Encoder-Velocity_Conversion (SubVI).vi"("delta  Encoder Count"=w402, "dt (uSec)"=w400) -> ("Rotational Velocity (RPS)"=w397:dbl)  [unwired: 7 in, 2 out]
        "RM Linear Velocity (rot/s)" <- w397
        n171 = call "Encoder-Velocity_Conversion (SubVI).vi"("delta  Encoder Count"=w401, "dt (uSec)"=w400) -> ("Rotational Velocity (RPS)"=w398:dbl)  [unwired: 7 in, 2 out]
        "RF Linear Velocity (rot/s)" <- w398
        n172 = Bundle("Rotational Velocity (RPS)"=w396, "Rotational Velocity (RPS)"=w395, "Rotational Velocity (RPS)"=w394, "Rotational Velocity (RPS)"=w393, "Rotational Velocity (RPS)"=w397, "Rotational Velocity (RPS)"=w398) -> (→"Current Rot Velocity (rot/s)":T2)  [unwired: 1 in]
      }
    }
  }
